vi "Create Path.vi"(4 "File Format":T3, 6 "Folder Format":T1, 7 "Parent path":T2, 8 "error in (no error)":errorcluster, 10 "Current time":timestamp, 11 "Directory":string) -> (0 "error out":errorcluster, 3 "Path":path)   [LabVIEW 2017, in "File.lvlib"]
uses:
  File.lvlib
  Control/File Format.ctl
  Control/Parent path.ctl
  Control/Folder Format.ctl
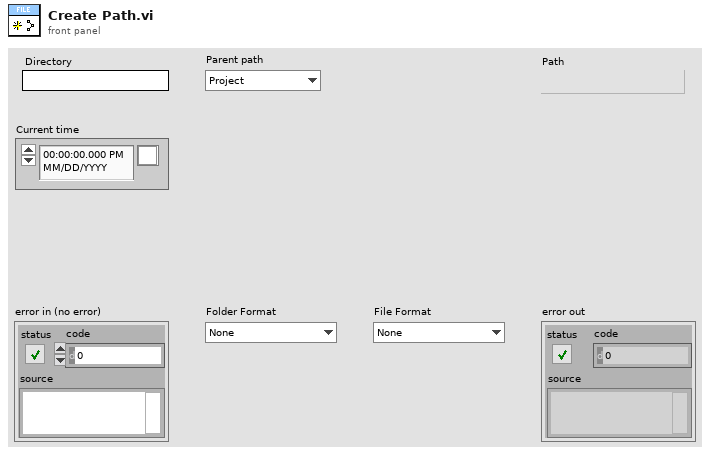
[diagram p1: front panel]
types:
  T1 = typedef "File.lvlib/Folder Format.ctl" = enum16{"None", "Folder Date", "Folder/Date"}
  T2 = typedef "File.lvlib/Parent path.ctl" = enum16{"Project", "Setting", "Log"}
  T3 = typedef "File.lvlib/File Format.ctl" = enum16{"None", "File Date", "File Time"}
  T4 = cluster{"Directory":string, "Folder":string, "Filename":string, "File type":string, "Date?":bool, "Time?":bool, "Path":path, "File Format":T3, "Current time":timestamp, "Parent path":T2, "Folder Format":T1}
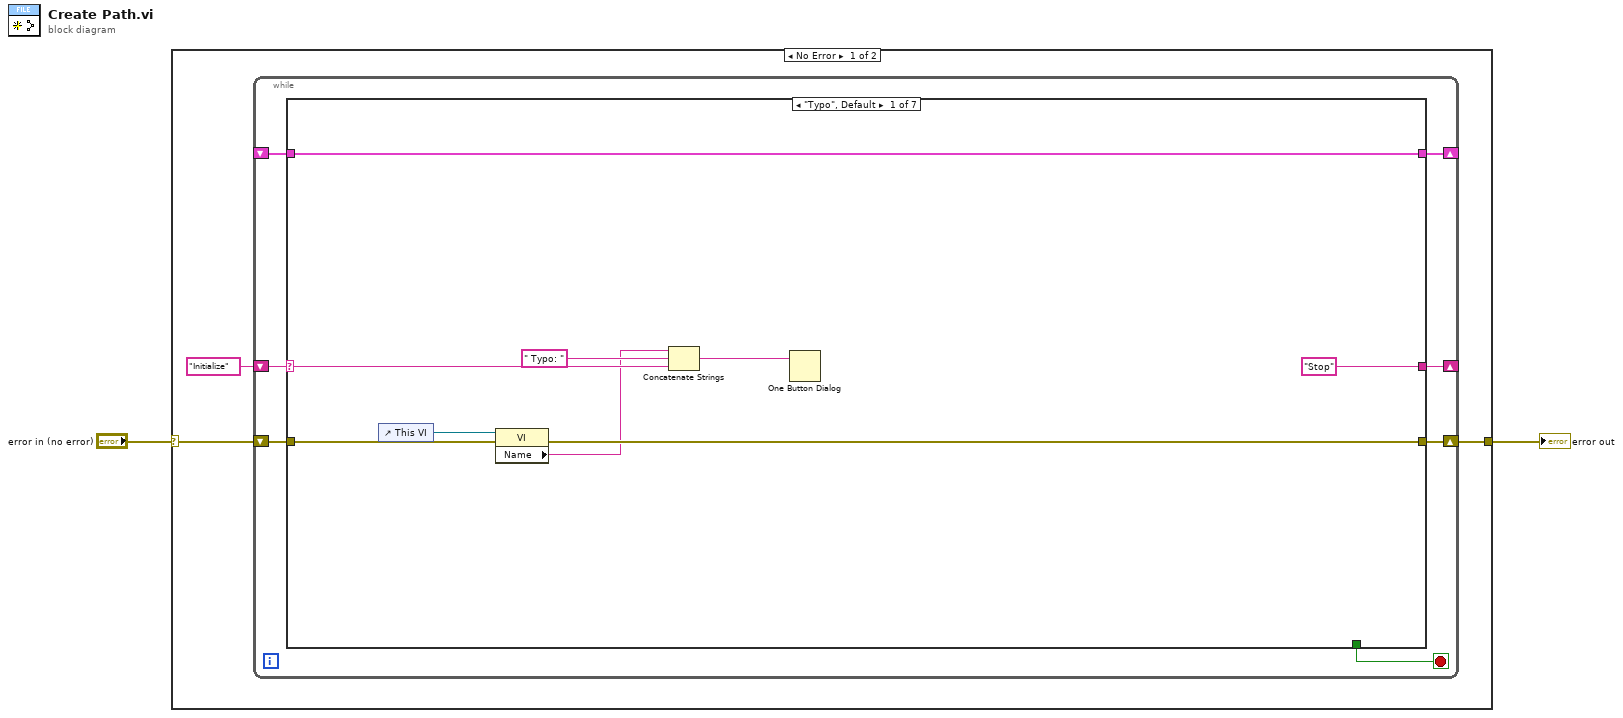
[diagram p0: block diagram]
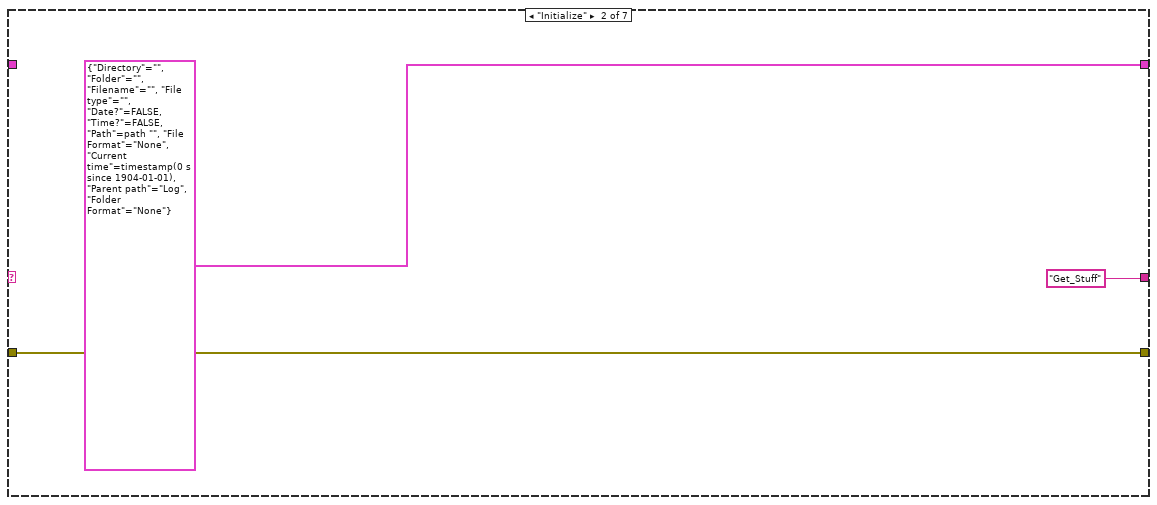
[diagram p2: hidden frame]
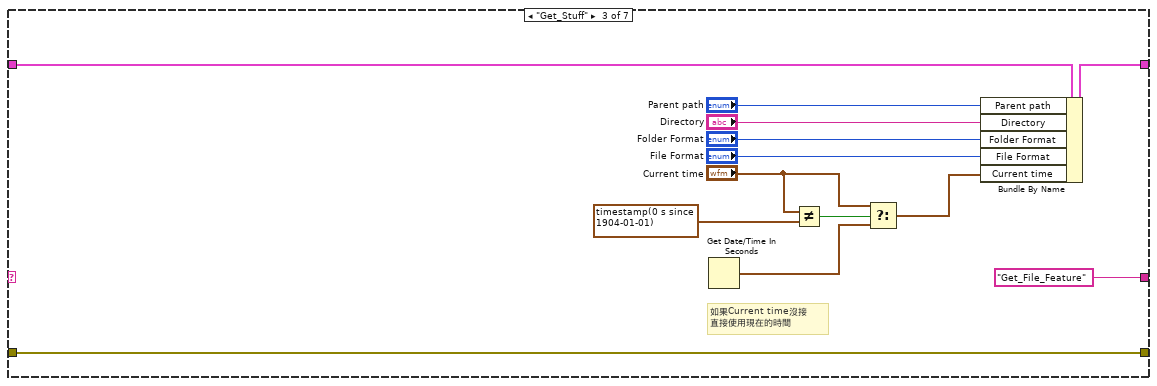
[diagram p3: hidden frame]
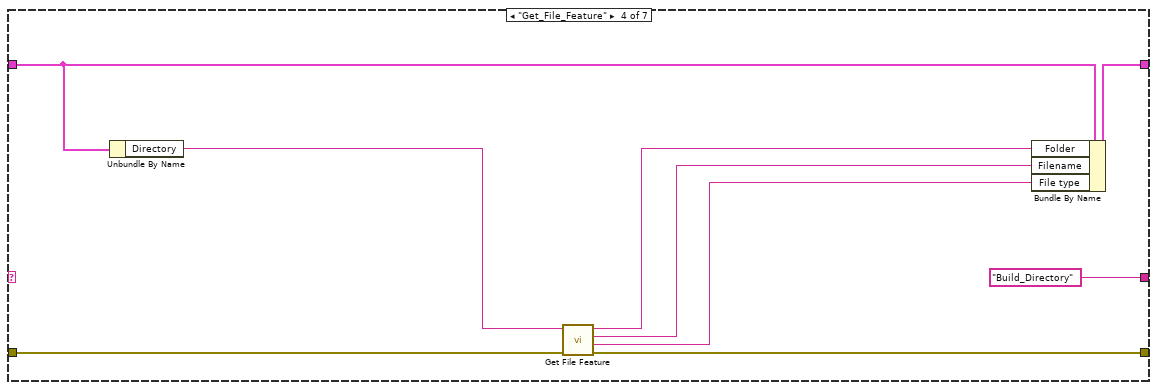
[diagram p4: hidden frame]
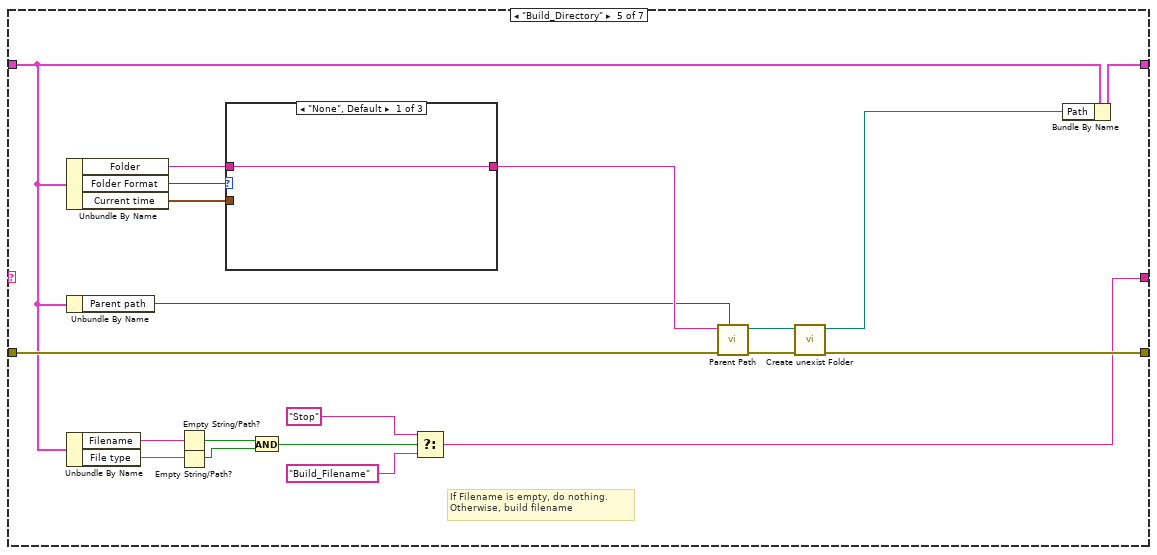
[diagram p5: hidden frame]
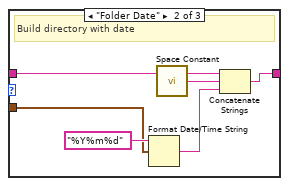
[diagram p6: hidden frame]
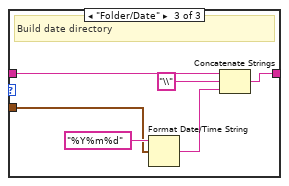
[diagram p7: hidden frame]
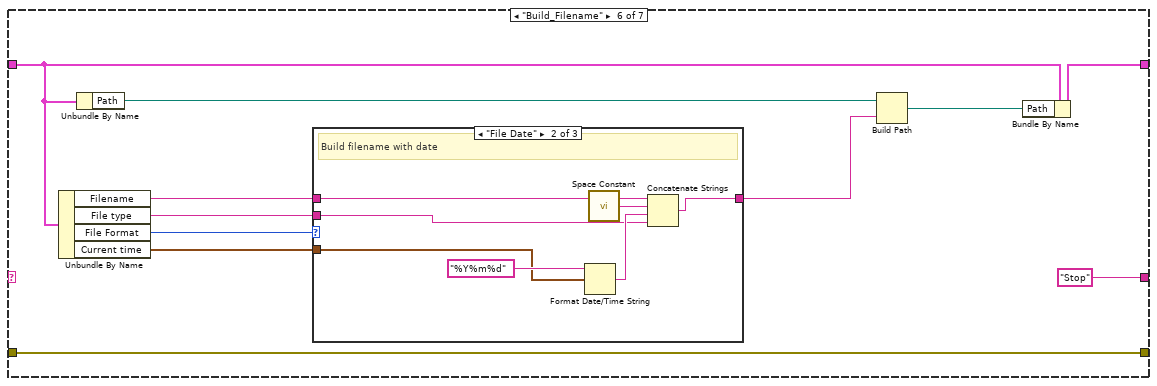
[diagram p8: hidden frame]
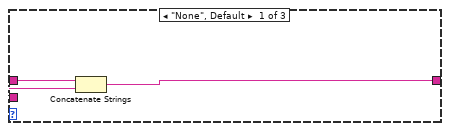
[diagram p9: hidden frame]
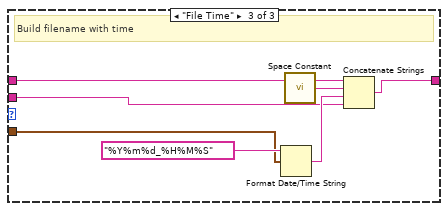
[diagram p10: hidden frame]
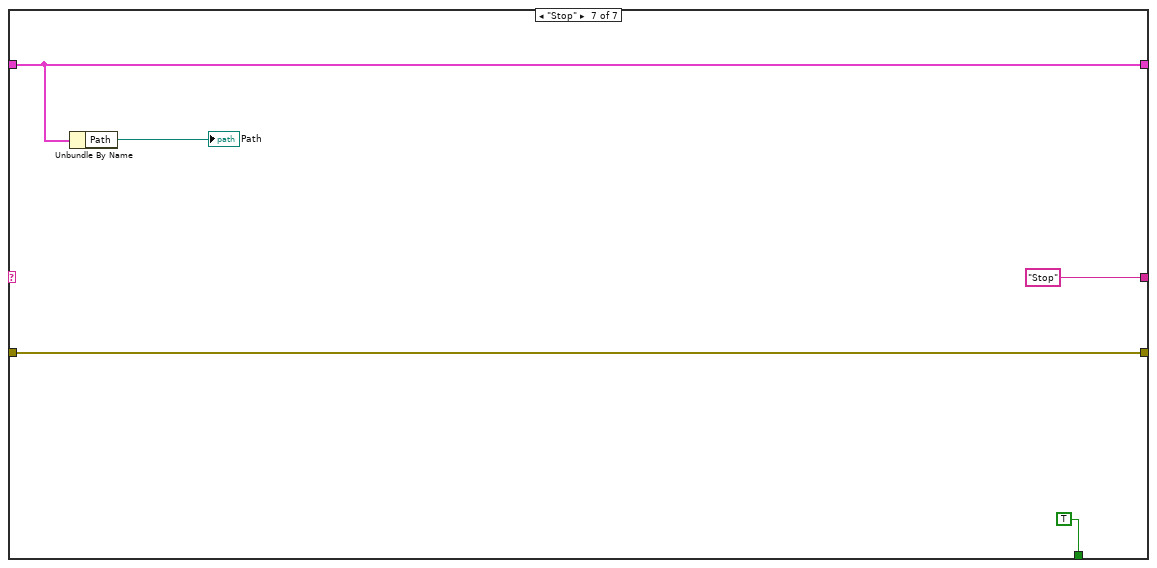
[diagram p11: hidden frame]
diagram:
  n1 = case shown="No Error" "error in (no error)" {
    selector: "error in (no error)" -> [w5 w113]
    tunnel: [w4 w113] -> w1
    frame No Error {
      n2 = while {
        shift-right: [w10] -> w4
        shift-left: w5 -> [w11]
        shift-right: [w9] -> _
        shift-left: "Initialize" -> [w12]
        shift-right: [w7] -> _
        shift-left: _ -> [w6]
        stop <- w8 stop-if-true
        n3 = case shown="\"Typo\", Default" w12 {
          selector: w12 -> [w18 _ _ _ _ _ _]
          tunnel: w11 -> [w21 w24 w33 w46 w66 w90 w112]
          tunnel: [w20 w24 w33 w45 w65 w90 w112] -> w10
          tunnel: ["Stop" "Get_Stuff" "Get_File_Feature" "Build_Directory" w58 "Stop" "Stop"] -> w9
          tunnel: [_ _ _ _ _ _ TRUE] -> w8
          tunnel: [w13 T4 {"Directory"="", "Folder"="", "Filename"="", "File type"="", "Date?"=FALSE, "Time?"=FALSE, "Path"=path "", "File Format"=enum."None", "Current time"=timestamp(0 s since 1904-01-01), "Parent path"=enum."Log", "Folder Format"=enum."None"} w36 w42 w63 w84 w109] -> w7
          tunnel: w6 -> [w13 _ w37 w44 w48 w87 w109]
          frame "Typo", Default {
            n4 = control-ref of="This VI"() -> (w19:refnum<vi>)
            n5 = property class="VI"(reference=w19, error in=w21) -> (error out=w20:errorcluster, "Name"=w16:string)  [unwired: 1 out]
            n6 = Concatenate Strings(w16, " Typo: ", w18) -> (w15:string)
            n7 = One Button Dialog(message=w15) -> ()  [unwired: 1 in, 1 out]
          }
          frame "Initialize" {
          }
          frame "Get_Stuff" {
            # "如果Current time沒接\n直接使用現在的時間"
            n8 = Get Date/Time In Seconds() -> (seconds since 1Jan1904=w27:timestamp)
            n9 = Not Equal?(x="Current time", y=timestamp(0 s since 1904-01-01)) -> (x != y?=w30:bool)
            n10 = Select(t="Current time", s=w30, f=w27) -> (s? t:f=w28:timestamp)
            n11 = Bundle By Name(cluster=w37, "Parent path"="Parent path", "Directory"="Directory", "Folder Format"="Folder Format", "File Format"="File Format", "Current time"=w28) -> (w36:T4)
          }
          frame "Get_File_Feature" {
            n12 = Unbundle By Name(w44) -> ("Directory"=w43:string)
            n13 = call "Get File Feature.vi"("error in (no error)"=w46, "String"=w43) -> ("error out"=w45:errorcluster, "File type"=w39:string, "Filename"=w40:string, "Folder"=w41:string)  [unwired: 6 in]
            n14 = Bundle By Name(cluster=w44, "Folder"=w41, "Filename"=w40, "File type"=w39) -> (w42:T4)
          }
          frame "Build_Directory" {
            # "If Filename is empty, do nothing.\nOtherwise, build filename"
            n15 = Unbundle By Name(w48) -> ("Folder"=w64:string, "Folder Format"=w57:T1, "Current time"=w49:timestamp)
            n16 = Unbundle By Name(w48) -> ("Parent path"=w47:T2)
            n17 = Unbundle By Name(w48) -> ("Filename"=w61:string, "File type"=w53:string)
            n18 = Empty String/Path?(string/path=w61) -> (empty?=w52:bool)
            n19 = Empty String/Path?(string/path=w53) -> (empty?=w51:bool)
            n20 = case shown="\"None\", Default" w57 {
              tunnel: w64 -> [w67 w71 w77]
              tunnel: [w67 w70 w76] -> w54
              tunnel: w49 -> [_ w68 w74]
              frame "None", Default {
              }
              frame "Folder Date" {
                # "Build directory with date"
                n21 = Format Date/Time String(time format string (%c)="%Y%m%d", seconds (now)=w68) -> (date/time string=w72:string)  [unwired: 1 in]
                n22 = call <vilib>:"Space Constant.vi"() -> ("String"=w69:string)
                n23 = Concatenate Strings(w71, w69, w72) -> (w70:string)
              }
              frame "Folder/Date" {
                # "Build date directory"
                n24 = Format Date/Time String(time format string (%c)="%Y%m%d", seconds (now)=w74) -> (date/time string=w78:string)  [unwired: 1 in]
                n25 = Concatenate Strings(w77, "\\", w78) -> (w76:string)
              }
            }
            n26 = And(x=w52, y=w51) -> (x .and. y?=w50:bool)
            n27 = Select(t="Stop", s=w50, f="Build_Filename") -> (s? t:f=w58:string)
            n28 = call "Parent Path.vi"("Parent path"=w47, "error in (no error)"=w66, "Path in"=w54) -> ("error out"=w56:errorcluster, "Path out"=w55:path)  [unwired: 7 in]
            n29 = call "Create unexist Folder.vi"("error in (no error)"=w56, "Path"=w55) -> ("error out"=w65:errorcluster, "Path Out"=w62:path)  [unwired: 8 in]
            n30 = Bundle By Name(cluster=w48, "Path"=w62) -> (w63:T4)
          }
          frame "Build_Filename" {
            n31 = Unbundle By Name(w87) -> ("Filename"=w89:string, "File type"=w88:string, "File Format"=w81:T3, "Current time"=w80:timestamp)
            n32 = Unbundle By Name(w87) -> ("Path"=w86:path)
            n33 = case shown="\"File Date\"" w81 {
              tunnel: w89 -> [w93 w100 w107]
              tunnel: w88 -> [w92 w97 w104]
              tunnel: [w91 w98 w105] -> w85
              tunnel: w80 -> [_ w94 w101]
              frame "None", Default {
                n34 = Concatenate Strings(w93, w92) -> (w91:string)
              }
              frame "File Date" {
                # "Build filename with date"
                n35 = Format Date/Time String(time format string (%c)="%Y%m%d", seconds (now)=w94) -> (date/time string=w99:string)  [unwired: 1 in]
                n36 = call <vilib>:"Space Constant.vi"() -> ("String"=w96:string)
                n37 = Concatenate Strings(w100, w96, w99, w97) -> (w98:string)
              }
              frame "File Time" {
                # "Build filename with time"
                n38 = Format Date/Time String(time format string (%c)="%Y%m%d_%H%M%S", seconds (now)=w101) -> (date/time string=w106:string)  [unwired: 1 in]
                n39 = call <vilib>:"Space Constant.vi"() -> ("String"=w103:string)
                n40 = Concatenate Strings(w107, w103, w106, w104) -> (w105:string)
              }
            }
            n41 = Build Path(base path=w86, name or relative path=w85) -> (appended path=w83:path)
            n42 = Bundle By Name(cluster=w87, "Path"=w83) -> (w84:T4)
          }
          frame "Stop" {
            n43 = Unbundle By Name(w109) -> ("Path"=→"Path":path)
          }
        }
      }
    }
    frame Error {
    }
  }
  "error out" <- w1
